vi "UI Update.vi"(8 "error in (no error)":errorcluster, 11 "Controller in":refnum<class "Controller.lvclass">) -> (0 "error out":errorcluster, 3 "Controller out":refnum<class "Controller.lvclass">)   [LabVIEW 2013, in "SET Project Editor.lvlib" / "Controller.lvclass"]
uses:
  Controller.lvclass
  Controller.lvclass/Controller.ctl
  SET Project Data/Project Data Class/Project Data.lvclass
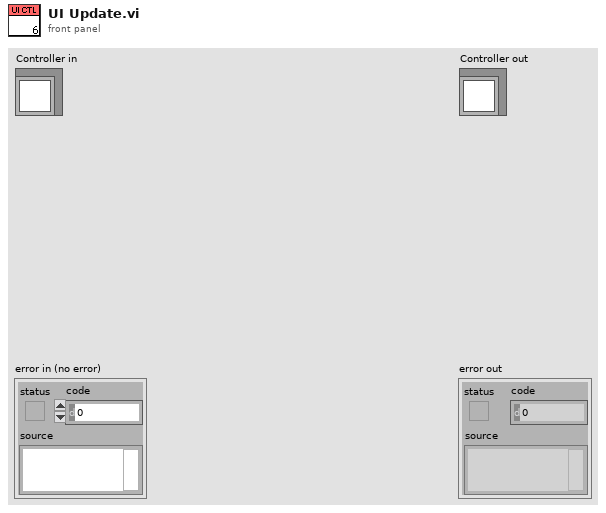
[diagram p1: front panel]
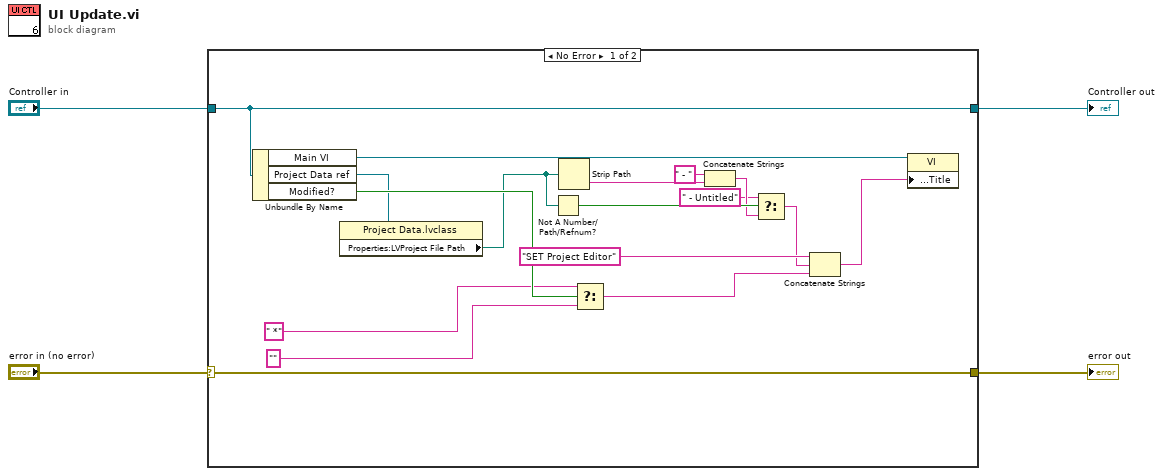
[diagram p0: block diagram]
diagram:
  n1 = case shown="No Error" "error in (no error)" {
    selector: "error in (no error)" -> [w21 w23]
    tunnel: [w21 w23] -> w2
    tunnel: [w20 w22] -> w3
    tunnel: "Controller in" -> [w20 w22]
    frame No Error {
      n2 = Unbundle By Name(w20) -> ("Main VI"=w19:refnum<vi>, "Project Data ref"=w6:refnum<data-value>, "Modified?"=w17:bool)
      n3 = property class="Project Data.lvclass"(reference=w6) -> ("Properties:LVProject File Path"=w5:path)  [unwired: 1 in, 2 out]
      n4 = Not A Number/Path/Refnum?(number/path/refnum=w5) -> (NaN/Path/Refnum?=w10:bool)
      n5 = Strip Path(path=w5) -> (name=w12:string)  [unwired: 1 out]
      n6 = Select(t=" *", s=w17, f="") -> (s? t:f=w13:string)
      n7 = Concatenate Strings(" - " ("string"), w12) -> (w9:string)
      n8 = Select(t=" - Untitled", s=w10, f=w9) -> (s? t:f=w7:string)
      n9 = Concatenate Strings("SET Project Editor", w7, w13) -> (w14:string)
      n10 = property class="VI"(reference=w19, "Front Panel.Title"=w14) -> ()  [unwired: 1 in, 2 out]
    }
    frame Error {
    }
  }
  "error out" <- w2
  "Controller out" <- w3
